vi "PLC OPC Datasocket Simulation Panel.vi"() -> ()   [LabVIEW 2013]
panel:
  in  "Invalid S No":dbl
  in  "Rerun":dbl
  in  "Station #":dbl
  in  "Last Test Result":dbl
  in  "Part Flange Size":dbl
  in  "Part Disp Size":dbl
  in  "Part Adapter Size":dbl
  in  "New Part?":dbl
  in  "Scan Trigger":dbl
  in  "Stop  Test":dbl
  in  "Start Test":dbl
  in  "Task Ready For Robot":dbl
  in  "Robot Available":dbl
  in  "Stop":bool
  # "Write Tags\nPC Writes to PLC\nPLC can only read these tags"
  # "Read Tags\nPC Reads from PLC"
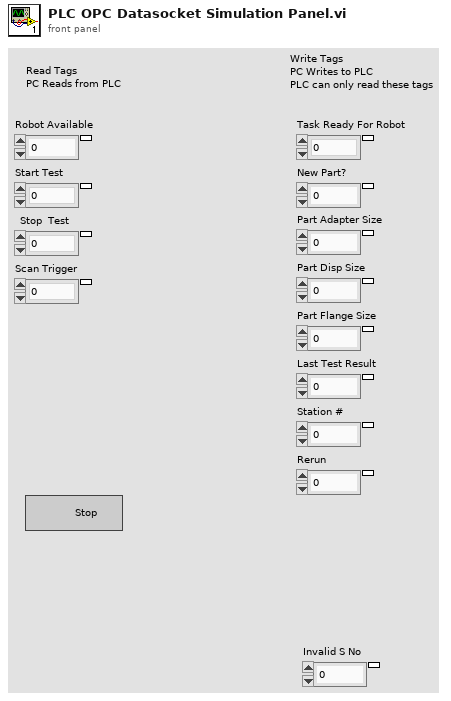
[diagram p1: front panel]
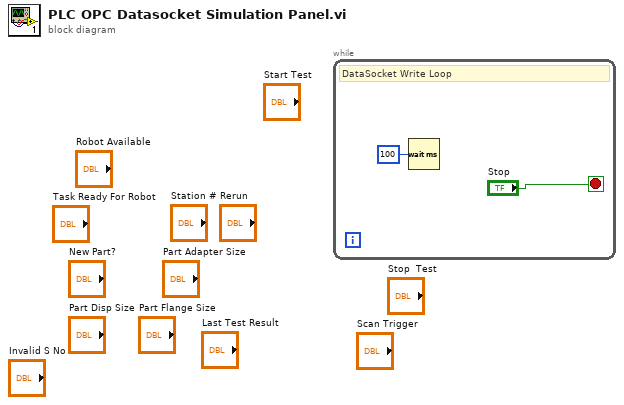
[diagram p0: block diagram]
diagram:
  n1 = while {
    stop <- "Stop" stop-if-true
    # "DataSocket Write Loop"
    n2 = Wait (ms)(milliseconds to wait=u32 100) -> ()  [unwired: 1 out]
  }
